vi "Coerce_Angle.vi"(11 "In Angle":dbl=2.1 format="%#_13g") -> (3 "Out Angle":dbl)   [LabVIEW 2014]
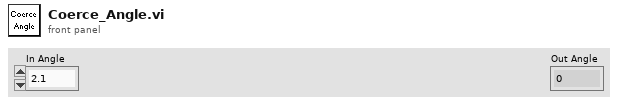
[diagram p1: front panel]
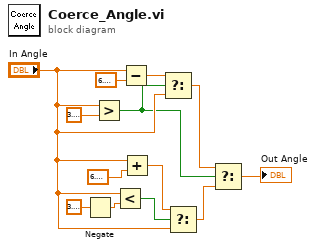
[diagram p0: block diagram]
diagram:
  n1 = Negate(x=3.141592653589793 ("y")) -> (-x=w9:dbl)
  n2 = Greater?(x="In Angle", y=3.141592653589793) -> (0:w4:bool)
  n3 = Less?(x="In Angle", y=w9) -> (x < y?=w6:bool)
  n4 = Subtract(x="In Angle", y=6.283185307179586) -> (x-y=w11:dbl)
  n5 = Add(x="In Angle", y=6.283185307179586) -> (x+y=w7:dbl)
  n6 = Select(t=w11, s=w4, f="In Angle") -> (s? t:f=w3:dbl)
  n7 = Select(t=w7, s=w6, f="In Angle") -> (s? t:f=w2:dbl)
  n8 = Select(t=w3, s=w4, f=w2) -> (s? t:f=→"Out Angle":dbl)
